vi "Init.vi"(10 "Queue":refnum<class "Queue.lvclass">) -> (3 "Last Ack Queue Msg Strategy out":refnum<class "Last Ack Queue Msg Strategy.lvclass">)   [LabVIEW 2021, in "jettl.lvlib" / "jettl Msg Last Ack Queue.lvlib" / "Last Ack Queue Msg Strategy.lvclass"]
uses:
  Last Ack Queue Msg Strategy.lvclass
  Queue/Queue.lvclass
  Last Ack Queue Msg Strategy.lvclass/Last Ack Queue Msg Strategy.ctl
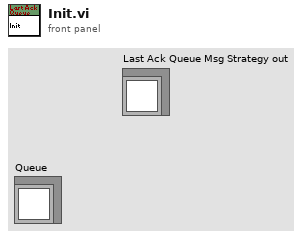
[diagram p1: front panel]
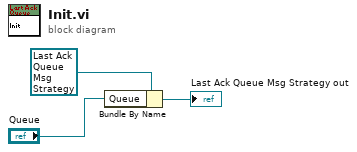
[diagram p0: block diagram]
diagram:
  n1 = Bundle By Name(cluster=refnum<class "Last Ack Queue Msg Strategy.lvclass"> refnum ("Last Ack Msg in"), "Queue"="Queue") -> (→"Last Ack Queue Msg Strategy out":refnum<class "Last Ack Queue Msg Strategy.lvclass">)
